vi "mai_chong_chan_sheng-5.12.vi"(0 "error in":errorcluster) -> (2 "error out":errorcluster)   [LabVIEW 2015]
uses:
  <vilib>/DAQmx/create/channels.llb/DAQmx Create Channel (CO-Pulse Generation-Frequency).vi
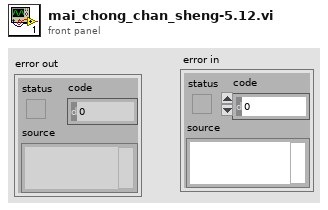
[diagram p1: front panel]
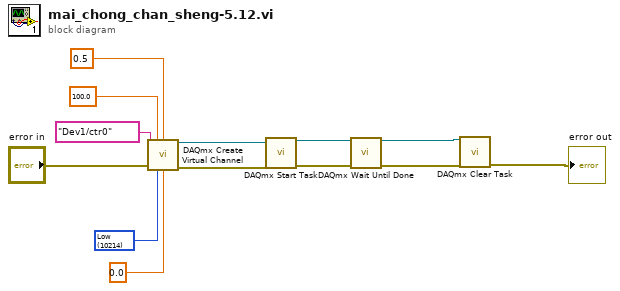
[diagram p0: block diagram]
diagram:
  w5 = 10214 items=["High"=10192, "Low"=10214] ("idle state")
  n1 = call-poly <vilib>:"DAQmx Create Virtual Channel.vi"("frequency"=100.0, "duty cycle"=0.5, "counter"=tag "Dev1/ctr0", "error in"="error in", "idle state"=w5, "initial delay"=0.0) -> ("task out"=w11:refnum<k21>, "error out"=w10:errorcluster)  [unwired: 8 in]
  n2 = call <vilib>:"DAQmx Start Task.vi"("task/channels in"=w11, "error in"=w10) -> ("task out"=w9:refnum<k21>, "error out"=w8:errorcluster)  [unwired: 12 in]
  n3 = call <vilib>:"DAQmx Wait Until Done.vi"("task/channels in"=w9, "error in"=w8) -> ("task out"=w7:refnum<k21>, "error out"=w6:errorcluster)  [unwired: 12 in]
  n4 = call <vilib>:"DAQmx Clear Task.vi"("task in"=w7, "error in"=w6) -> ("error out"=→"error out":errorcluster)  [unwired: 13 in]
